vi "Attenuator Handle Test Complete.vi"(6 "Quick Mode (F)":bool, 8 "error in (no error)":errorcluster, 9 "Test Parameters":T1={"Stimulus"={"ATT Stimulus"={"Normalize"=TRUE, "Value (dB)"=0.0}, "VNA Stimulus"={"Use Instrument Settings"=FALSE, "Blank Frequencies"=FALSE, "Sweep Type"=enum."Linear", "Sweep"={"Fstart"=500.0, "Fstop"=1500.0, "Units"=enum."MHz", "Points"=201}, "Power (dBm)"=999.0, "IFBW (Hz)"=-1.0, "Sweep Time (s)"=-1.0, "Calibration"={"State"=FALSE, "String"=""}}}, "Measurement"={"Step (dB)"=enum."0.25", "Start (dB)"=0.0, "Stop (dB)"=31.75}, "Limit"={"Maximum Error"=0.3}, "Normalization"={"Normalized?"=FALSE, "Normalization Values (dB)"=[]}} {"Stimulus"."VNA Stimulus"."Sweep Time (s)" format="%.3g"}, 10 "Done?":bool, 11 "Queue":refnum<queue>) -> (0 "error out":errorcluster)   [LabVIEW 2011]
uses:
  TypeDefs/Attenuator Queue Cluster.ctl
  TypeDefs/Attenuator Test Parameters.ctl
  TypeDefs/Attenuator Stimulus Parameters.ctl
  TypeDefs/Attenuator ATT Stimulus.ctl
  TypeDefs/Attenuator VNA Stimulus.ctl
  S Parameter/TypeDefs/SP Frequency Units.ctl
  TypeDefs/Attenuator VNA Calibration State.ctl
  TypeDefs/Attenuator Measurement Cluster.ctl
  TypeDefs/Attenuator Limit.ctl
  TypeDefs/Attenuator Calibration State.ctl
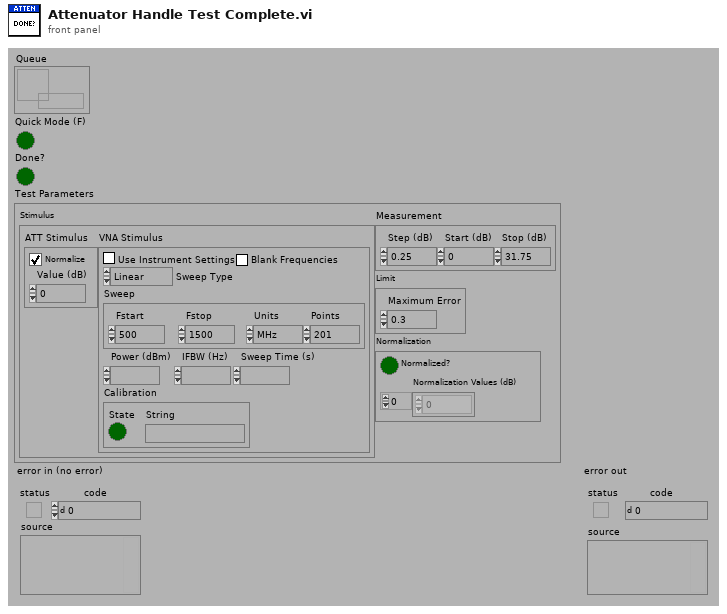
[diagram p1: front panel]
types:
  T1 = typedef "Attenuator Test Parameters.ctl" = cluster{"Stimulus":T2, "Measurement":T7, "Limit":T8, "Normalization":T9}
  T2 = typedef "Attenuator Stimulus Parameters.ctl" = cluster{"ATT Stimulus":T3, "VNA Stimulus":T4}
  T3 = typedef "Attenuator ATT Stimulus.ctl" = cluster{"Normalize":bool, "Value (dB)":dbl}
  T4 = typedef "Attenuator VNA Stimulus.ctl" = cluster{"Use Instrument Settings":bool, "Blank Frequencies":bool, "Sweep Type":enum32{"Linear", "Logarithmic", "List", "Power", "CW"}, "Sweep":cluster{"Fstart":dbl, "Fstop":dbl, "Units":T5, "Points":i32}, "Power (dBm)":dbl, "IFBW (Hz)":dbl, "Sweep Time (s)":dbl, "Calibration":T6}
  T5 = typedef "SP Frequency Units.ctl" = enum16{"Hz", "kHz", "MHz", "GHz", "Points"}
  T6 = typedef "Attenuator VNA Calibration State.ctl" = cluster{"State":bool, "String":string}
  T7 = typedef "Attenuator Measurement Cluster.ctl" = cluster{"Step (dB)":enum16{"0.25", "0.50", "1.00"}, "Start (dB)":dbl, "Stop (dB)":dbl}
  T8 = typedef "Attenuator Limit.ctl" = cluster{"Maximum Error":dbl}
  T9 = typedef "Attenuator Calibration State.ctl" = cluster{"Normalized?":bool, "Normalization Values (dB)":dbl[]}
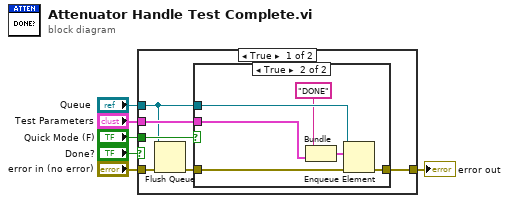
[diagram p0: block diagram]
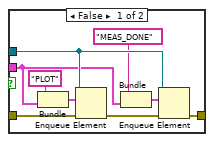
[diagram p2: hidden frame]
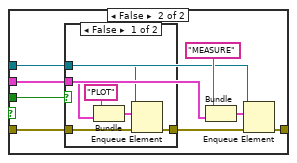
[diagram p3: hidden frame]
diagram:
  n1 = case shown="True" "Done?" {
    tunnel: [w12 w31] -> w6
    tunnel: "Queue" -> [w8 w29]
    tunnel: "error in (no error)" -> [w9 w35]
    tunnel: "Test Parameters" -> [w11 w28]
    tunnel: "Quick Mode (F)" -> [w10 w34]
    frame True {
      n2 = Flush Queue(queue=w8, error in (no error)=w9) -> (error out=w7:errorcluster)  [unwired: 2 out]
      n3 = case shown="True" w10 {
        tunnel: [w17 w27] -> w12
        tunnel: w8 -> [w16 w25]
        tunnel: w7 -> [w13 w22]
        tunnel: w11 -> [w15 w24]
        frame False {
          n4 = Bundle("PLOT", "Test Parameters"=w15) -> (w20:cluster{string, "Test Parameters":T1})  [unwired: 1 out]
          n5 = Enqueue Element(queue=w16, element=w20, error in (no error)=w13) -> (error out=w18:errorcluster)  [unwired: 3 out]
          n6 = Bundle("MEAS_DONE", "Test Parameters"=w15) -> (w19:cluster{string, "Test Parameters":T1})  [unwired: 1 out]
          n7 = Enqueue Element(queue=w16, element=w19, error in (no error)=w18) -> (error out=w17:errorcluster)  [unwired: 3 out]
        }
        frame True {
          n8 = Bundle("DONE", "Test Parameters"=w24) -> (w26:cluster{string, "Test Parameters":T1})  [unwired: 1 out]
          n9 = Enqueue Element(queue=w25, element=w26, error in (no error)=w22) -> (error out=w27:errorcluster)  [unwired: 3 out]
        }
      }
    }
    frame False {
      n10 = case shown="False" w34 {
        tunnel: [w36 w42] -> w32
        tunnel: w29 -> [w39 _]
        tunnel: w35 -> [w37 w42]
        tunnel: w28 -> [w38 _]
        frame False {
          n11 = Bundle("PLOT", "Test Parameters"=w38) -> (w40:cluster{string, "Test Parameters":T1})  [unwired: 1 out]
          n12 = Enqueue Element(queue=w39, element=w40, error in (no error)=w37) -> (error out=w36:errorcluster)  [unwired: 3 out]
        }
        frame True {
        }
      }
      n13 = Bundle("MEASURE", "Test Parameters"=w28) -> (w30:cluster{string, "Test Parameters":T1})  [unwired: 1 out]
      n14 = Enqueue Element(queue=w29, element=w30, error in (no error)=w32) -> (error out=w31:errorcluster)  [unwired: 3 out]
    }
  }
  "error out" <- w6
